vi "face rotate F-.vi"(8 "error in (no error)":errorcluster, 11 "cube in":T1) -> (0 "error out":errorcluster, 3 "cube out":T1)   [LabVIEW 2011]
uses:
  Typedef/cube.ctl
  Typedef/face.ctl
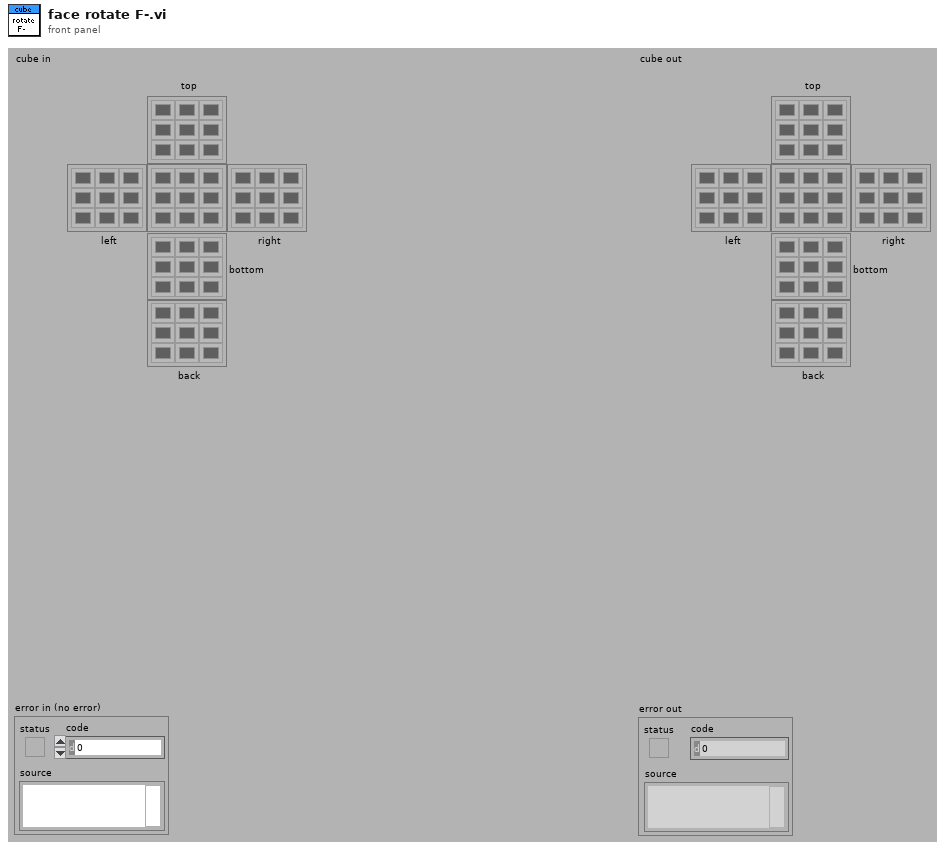
[diagram p1: front panel]
types:
  T1 = typedef "cube.ctl" = cluster{"top":T2, "left":T2, "right":T2, "bottom":T2, "back":T2, "front":T2}
  T2 = typedef "face.ctl" = u32[][]
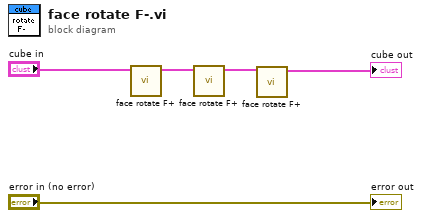
[diagram p0: block diagram]
diagram:
  n1 = call "face rotate F+.vi"("cube in"="cube in") -> ("cube out"=w3:T1)  [unwired: 9 in, 1 out]
  n2 = call "face rotate F+.vi"("cube in"=w3) -> ("cube out"=w2:T1)  [unwired: 9 in, 1 out]
  n3 = call "face rotate F+.vi"("cube in"=w2) -> ("cube out"=→"cube out":T1)  [unwired: 9 in, 1 out]
  "error out" <- "error in (no error)"
